vi "convertErrorIntToText.vi"(1 "Error Int In (function return)":u32, 2 "Error String In":string) -> (0 "Error String Out":string)   [LabVIEW 2021]
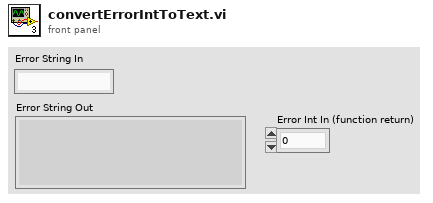
[diagram p1: front panel]
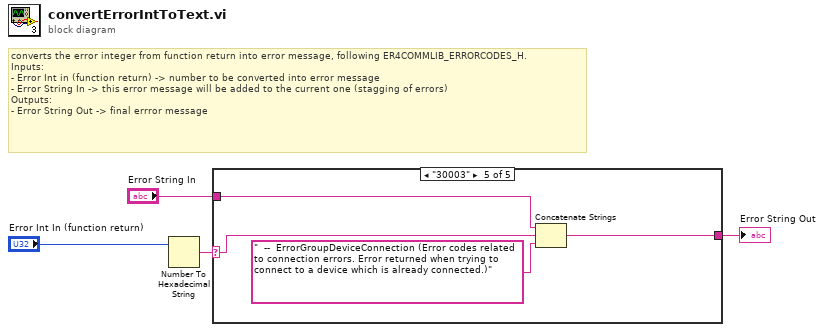
[diagram p0: block diagram]
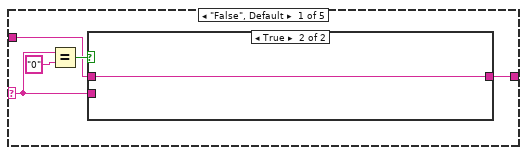
[diagram p2: hidden frame]
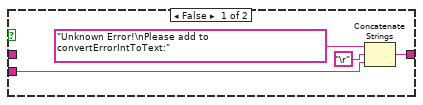
[diagram p3: hidden frame]
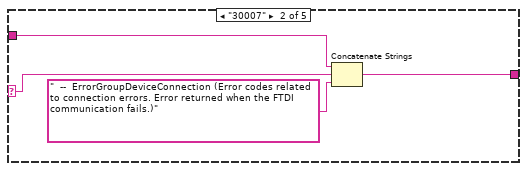
[diagram p4: hidden frame]
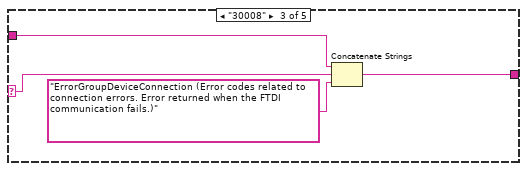
[diagram p5: hidden frame]
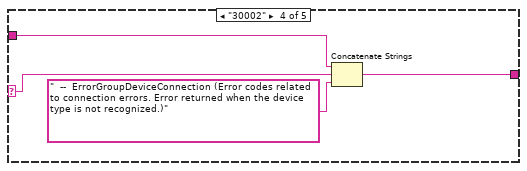
[diagram p6: hidden frame]
diagram:
  # "converts the error integer from function return into error message, following ER4COMMLIB_ERRORCODES_H.\nInputs: \n- Error Int in (function return) -> number to be converted into error message\n- Error String In -> this error message will be added to the current one (stagging of errors)\nOutputs:\n- Error String Out -> final errror message"
  n1 = Number To Hexadecimal String(2:"Error Int In (function return)") -> (0:w2:string)  [unwired: 1 in]
  n2 = case shown="\"30003\"" w2 {
    selector: w2 -> [w6 w16 w19 w23 w27]
    tunnel: [w8 w17 w21 w25 w29] -> w3
    tunnel: "Error String In" -> [w5 w15 w20 w24 w28]
    frame "False", Default {
      n3 = Equal?(x=w6, y="0") -> (x = y?=w7:bool)
      n4 = case shown="True" w7 {
        tunnel: w5 -> [_ w14]
        tunnel: [w12 w14] -> w8
        tunnel: w6 -> [w11 _]
        frame False {
          n5 = Concatenate Strings("Unknown Error!\nPlease add to convertErrorIntToText:", "\r", w11) -> (w12:string)
        }
        frame True {
        }
      }
    }
    frame "30007" {
      n6 = Concatenate Strings(w15, w16, "  --  ErrorGroupDeviceConnection (Error codes related to connection errors. Error returned when the FTDI communication fails.)") -> (w17:string)
    }
    frame "30008" {
      n7 = Concatenate Strings(w20, w19, "ErrorGroupDeviceConnection (Error codes related to connection errors. Error returned when the FTDI communication fails.)") -> (w21:string)
    }
    frame "30002" {
      n8 = Concatenate Strings(w24, w23, "  --  ErrorGroupDeviceConnection (Error codes related to connection errors. Error returned when the device type is not recognized.)") -> (w25:string)
    }
    frame "30003" {
      n9 = Concatenate Strings(w28, w27, "  --  ErrorGroupDeviceConnection (Error codes related to connection errors. Error returned when trying to connect to a device which is already connected.)") -> (w29:string)
    }
  }
  "Error String Out" <- w3
